vi "Positioner Control.vi"(6 "control_move_length":i64, 7 "control_positioner_reference":refnum<class "SA_CTL.lvclass">, 8 "mode":string, 9 "index":i64, 10 "control_move_direction":string, 11 "control_request":string) -> (0 "indicator_positioner_ismoving_y":bool, 1 "indicator_positioner_ismoving_x":bool, 2 "indicator_positioner_status":bool, 3 "indicator_positioner_position":cluster{"x":i64, "y":i64, "z":i64}, 4 "indicator_positioner_ismoving_z":bool, 5 "indicator_positioner_reference":refnum<class "SA_CTL.lvclass">)   [LabVIEW 2020]
uses:
  <vilib>/SmarAct/SmarActCTL/SA_CTL.lvclass
panel:
  out "error out 4":errorcluster
  out "error out 3":errorcluster
  out "error out 2":errorcluster
  out "error out":errorcluster
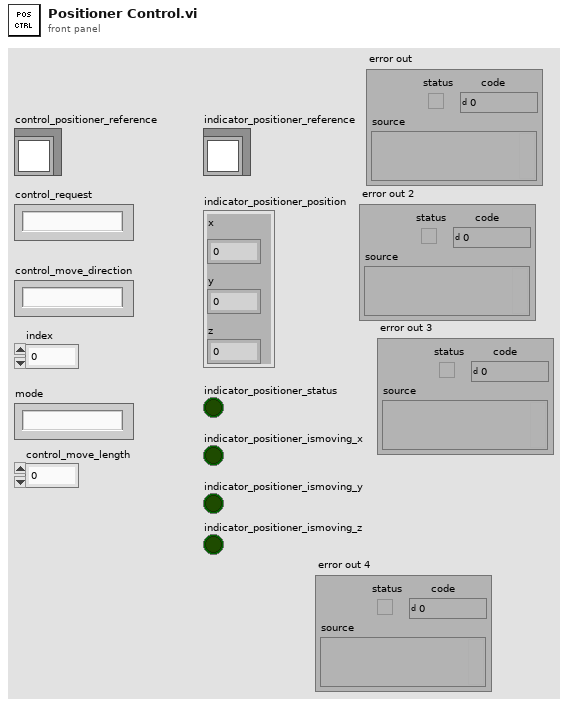
[diagram p1: front panel]
types:
  T1 = cluster{"Position":i64, "Position":i64, "Position":i64}
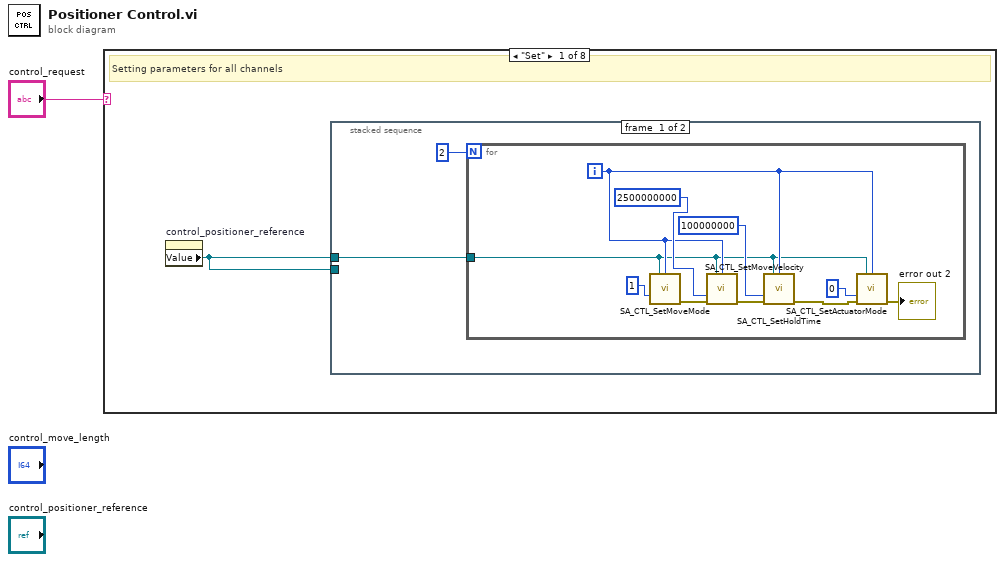
[diagram p0: block diagram]
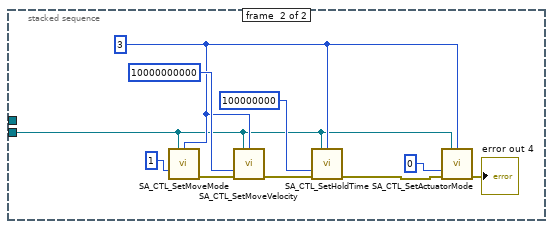
[diagram p2: hidden frame]
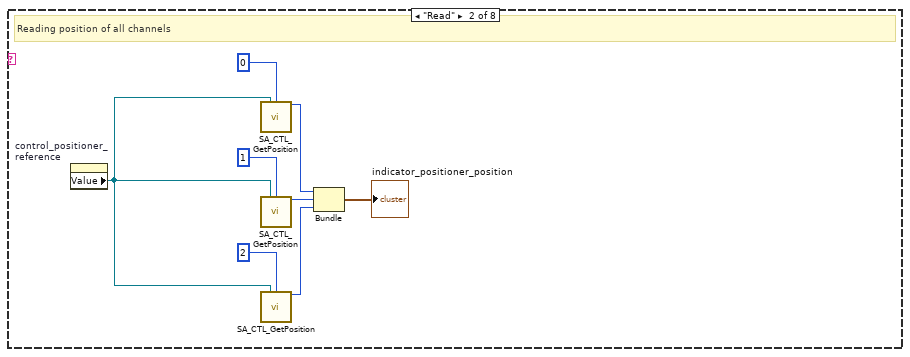
[diagram p3: hidden frame]
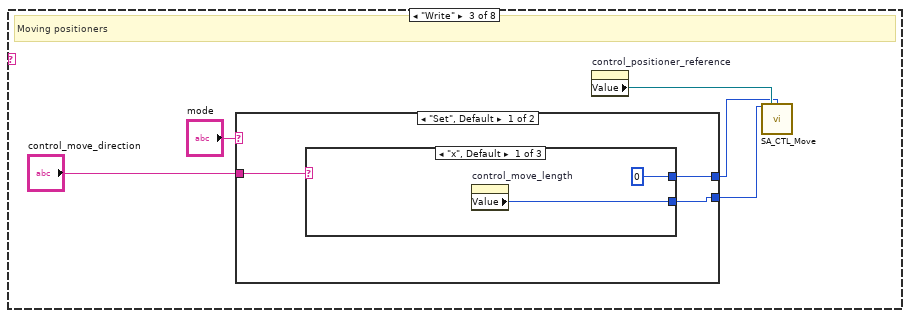
[diagram p4: hidden frame]
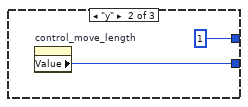
[diagram p5: hidden frame]
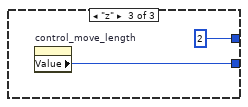
[diagram p6: hidden frame]
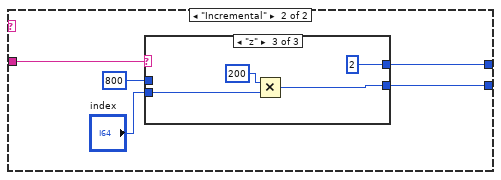
[diagram p7: hidden frame]
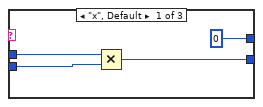
[diagram p8: hidden frame]
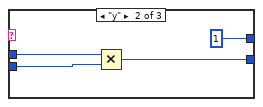
[diagram p9: hidden frame]
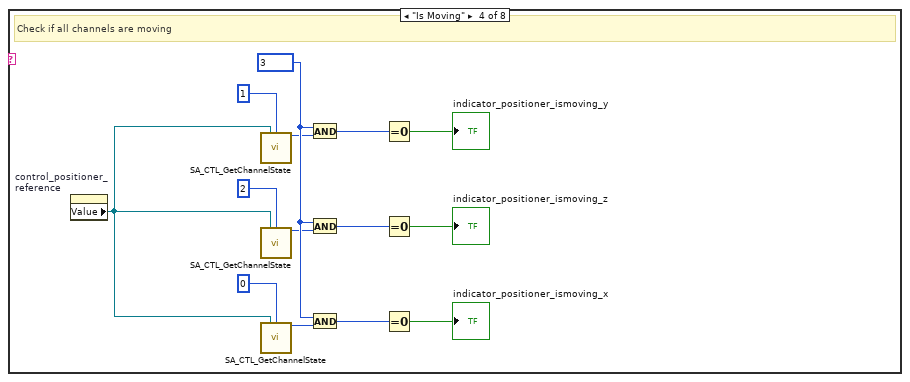
[diagram p10: hidden frame]
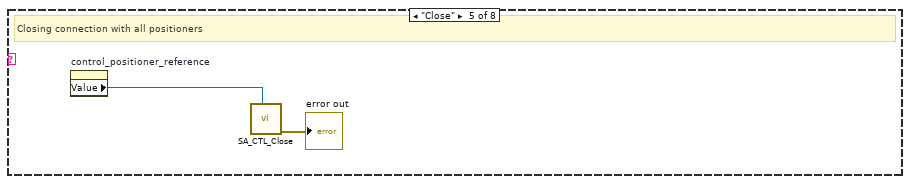
[diagram p11: hidden frame]
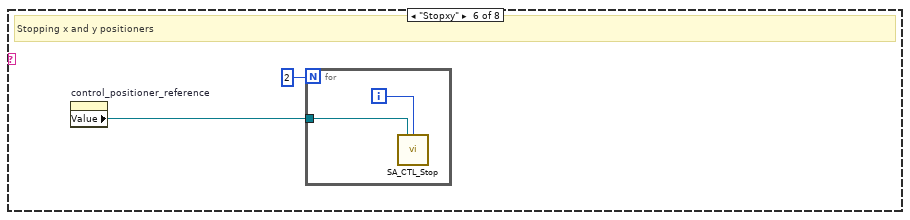
[diagram p12: hidden frame]
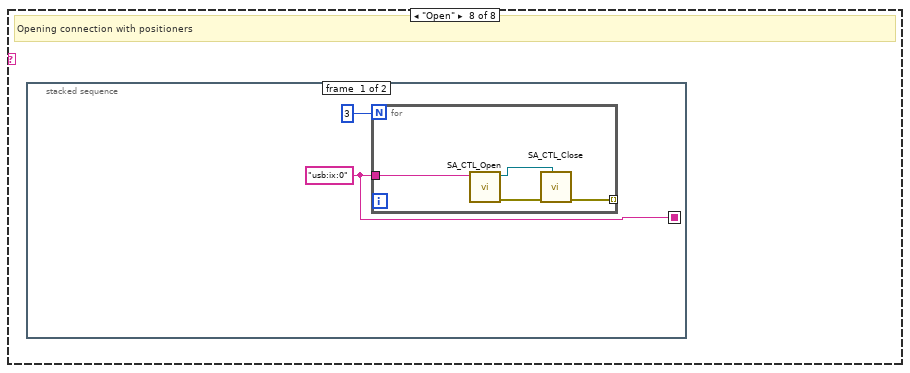
[diagram p14: hidden frame]
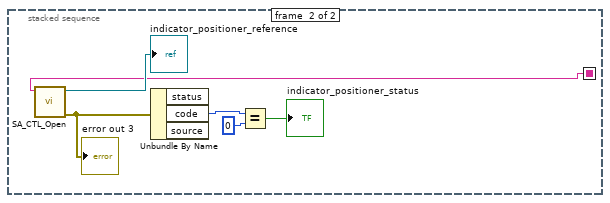
[diagram p15: hidden frame]
diagram:
  n1 = case shown="\"Set\"" "control_request" {
    frame "Set" {
      # "Setting parameters for all channels"
      n2 = property on="control_positioner_reference" class="LVClassControl (strict)"() -> ("Value"=w2:refnum<class "SA_CTL.lvclass">)  [unwired: 2 in, 2 out]
      n3 = stacked-sequence {
        tunnel: w2 -> [w3 _]
        tunnel: w2 -> [_ w16]
        frame #0 {
          n4 = for {
            N: 2 -> [_]
            tunnel: w3 -> [w5]
            i -> [w6]
            n5 = call <vilib>:"SA_CTL_SetMoveMode.vi"("SA_CTL_Handle"=w5, "channel"=w6, "MoveMode"=1) -> ("error out"=w12:errorcluster)  [unwired: 12 in]
            n6 = call <vilib>:"SA_CTL_SetMoveVelocity.vi"("SA_CTL_Handle"=w5, "channel"=w6, "MoveVelocity"=i64 2500000000 ("FindReferenceVelocity"), "error in (no error)"=w12) -> ("error out"=w11:errorcluster)  [unwired: 11 in]
            n7 = call <vilib>:"SA_CTL_SetHoldTime.vi"("SA_CTL_Handle"=w5, "channel"=w6, "HoldTime"=100000000, "error in (no error)"=w11) -> ("error out"=w9:errorcluster)  [unwired: 11 in]
            n8 = call <vilib>:"SA_CTL_SetActuatorMode.vi"("SA_CTL_Handle"=w5, "channel"=w6, "ActuatorMode"=0, "error in (no error)"=w9) -> ("error out"=→"error out 2":errorcluster)  [unwired: 11 in]
          }
        }
        frame #1 {
          w17 = 3 ("MoveMode")
          n9 = call <vilib>:"SA_CTL_SetMoveMode.vi"("SA_CTL_Handle"=w16, "channel"=w17, "MoveMode"=1) -> ("error out"=w22:errorcluster)  [unwired: 12 in]
          n10 = call <vilib>:"SA_CTL_SetMoveVelocity.vi"("SA_CTL_Handle"=w16, "channel"=w17, "MoveVelocity"=i64 10000000000 ("FindReferenceVelocity"), "error in (no error)"=w22) -> ("error out"=w21:errorcluster)  [unwired: 11 in]
          n11 = call <vilib>:"SA_CTL_SetHoldTime.vi"("SA_CTL_Handle"=w16, "channel"=w17, "HoldTime"=100000000, "error in (no error)"=w21) -> ("error out"=w19:errorcluster)  [unwired: 11 in]
          n12 = call <vilib>:"SA_CTL_SetActuatorMode.vi"("SA_CTL_Handle"=w16, "channel"=w17, "ActuatorMode"=0, "error in (no error)"=w19) -> ("error out"=→"error out 4":errorcluster)  [unwired: 11 in]
        }
      }
    }
    frame "Read" {
      # "Reading position of all channels"
      n13 = property on="control_positioner_reference" class="LVClassControl (strict)"() -> ("Value"=w32:refnum<class "SA_CTL.lvclass">)  [unwired: 2 in, 2 out]
      n14 = call <vilib>:"SA_CTL_GetPosition.vi"("SA_CTL_Handle"=w32, "channel"=i8 0) -> ("Position"=w28:i64)  [unwired: 12 in, 1 out]
      n15 = call <vilib>:"SA_CTL_GetPosition.vi"("SA_CTL_Handle"=w32, "channel"=i8 1) -> ("Position"=w27:i64)  [unwired: 12 in, 1 out]
      n16 = call <vilib>:"SA_CTL_GetPosition.vi"("SA_CTL_Handle"=w32, "channel"=i8 2) -> ("Position"=w26:i64)  [unwired: 12 in, 1 out]
      n17 = Bundle("Position"=w28, "Position"=w27, "Position"=w26) -> (→"indicator_positioner_position":T1)  [unwired: 1 in]
    }
    frame "Write" {
      # "Moving positioners"
      n18 = case shown="\"Set\", Default" "mode" {
        tunnel: "control_move_direction" -> [w40 w51]
        tunnel: [w38 w49] -> w35
        tunnel: [w39 w48] -> w34
        frame "Set", Default {
          n19 = case shown="\"x\", Default" w40 {
            tunnel: [w41 w43 w45] -> w38
            tunnel: [i8 0 ("channel") i8 1 ("channel") i8 2 ("channel")] -> w39
            frame "x", Default {
              n20 = property on="control_move_length" class="DigNum (strict)"() -> ("Value"=w41:i64)  [unwired: 2 in, 2 out]
            }
            frame "y" {
              n21 = property on="control_move_length" class="DigNum (strict)"() -> ("Value"=w43:i64)  [unwired: 2 in, 2 out]
            }
            frame "z" {
              n22 = property on="control_move_length" class="DigNum (strict)"() -> ("Value"=w45:i64)  [unwired: 2 in, 2 out]
            }
          }
        }
        frame "Incremental" {
          n23 = case shown="\"z\"" w51 {
            tunnel: "index" -> [w55 w59 w63]
            tunnel: [w54 w57 w61] -> w49
            tunnel: [i8 0 ("channel") i8 1 ("channel") i8 2 ("channel")] -> w48
            tunnel: i64 800 ("moveValue") -> [w52 w56 _]
            frame "x", Default {
              n24 = Multiply(x=w52, y=w55) -> (x*y=w54:i64)
            }
            frame "y" {
              n25 = Multiply(x=w56, y=w59) -> (x*y=w57:i64)
            }
            frame "z" {
              n26 = Multiply(x=i64 200, y=w63) -> (x*y=w61:i64)
            }
          }
        }
      }
      n27 = property on="control_positioner_reference" class="LVClassControl (strict)"() -> ("Value"=w36:refnum<class "SA_CTL.lvclass">)  [unwired: 2 in, 2 out]
      n28 = call <vilib>:"SA_CTL_Move.vi"("moveValue"=w35, "SA_CTL_Handle"=w36, "channel"=w34) -> ()  [unwired: 12 in, 1 out]
    }
    frame "Is Moving" {
      w70 = 3 ("Mask")
      # "Check if all channels are moving"
      n29 = property on="control_positioner_reference" class="LVClassControl (strict)"() -> ("Value"=w74:refnum<class "SA_CTL.lvclass">)  [unwired: 2 in, 2 out]
      n30 = call <vilib>:"SA_CTL_GetChannelState.vi"("SA_CTL_Handle"=w74, "channel"=i8 1) -> ("ChannelState"=w68:i32)  [unwired: 12 in, 1 out]
      n31 = call <vilib>:"SA_CTL_GetChannelState.vi"("SA_CTL_Handle"=w74, "channel"=i8 2) -> ("ChannelState"=w67:i32)  [unwired: 12 in, 1 out]
      n32 = call <vilib>:"SA_CTL_GetChannelState.vi"("SA_CTL_Handle"=w74, "channel"=i8 0) -> ("ChannelState"=w69:i32)  [unwired: 12 in, 1 out]
      n33 = And(x=w70, y=w68) -> (x .and. y?=w72:i32)
      n34 = And(x=w70, y=w67) -> (x .and. y?=w71:i32)
      n35 = And(x=w70, y=w69) -> (x .and. y?=w73:i32)
      n36 = Equal To 0?(x=w72) -> (x = 0?=→"indicator_positioner_ismoving_y":bool)
      n37 = Equal To 0?(x=w71) -> (x = 0?=→"indicator_positioner_ismoving_z":bool)
      n38 = Equal To 0?(x=w73) -> (x = 0?=→"indicator_positioner_ismoving_x":bool)
    }
    frame "Close" {
      # "Closing connection with all positioners"
      n39 = property on="control_positioner_reference" class="LVClassControl (strict)"() -> ("Value"=w79:refnum<class "SA_CTL.lvclass">)  [unwired: 2 in, 2 out]
      n40 = call <vilib>:"SA_CTL_Close.vi"("SA_CTL_Handle"=w79) -> ("error out"=→"error out":errorcluster)  [unwired: 10 in]
    }
    frame "Stopxy" {
      # "Stopping x and y positioners"
      n41 = property on="control_positioner_reference" class="LVClassControl (strict)"() -> ("Value"=w81:refnum<class "SA_CTL.lvclass">)  [unwired: 2 in, 2 out]
      n42 = for {
        N: 2 -> [_]
        tunnel: w81 -> [w83]
        i -> [w82]
        n43 = call <vilib>:"SA_CTL_Stop.vi"("SA_CTL_Handle"=w83, "channel"=w82) -> ()  [unwired: 13 in, 1 out]
      }
    }
    frame "Default", Default {
    }
    frame "Open" {
      # "Opening connection with positioners"
      n44 = stacked-sequence {
        seq-local: [w84 _] -> [_ w90]
        frame #0 {
          w84 = "usb:ix:0" ("locator")
          n45 = for {
            N: 3 -> [_]
            tunnel: w84 -> [w87]
            tunnel: [w86] -> _ mode=indexing
            n46 = call <vilib>:"SA_CTL_Open.vi"("locator"=w87) -> ("error out"=w88:errorcluster, "SA_CTL_Handle"=w89:refnum<class "SA_CTL.lvclass">)  [unwired: 9 in]
            n47 = call <vilib>:"SA_CTL_Close.vi"("SA_CTL_Handle"=w89, "error in (no error)"=w88) -> ("error out"=w86:errorcluster)  [unwired: 9 in]
          }
        }
        frame #1 {
          n48 = call <vilib>:"SA_CTL_Open.vi"("locator"=w90) -> ("error out"=w93:errorcluster, "SA_CTL_Handle"=→"indicator_positioner_reference":refnum<class "SA_CTL.lvclass">)  [unwired: 9 in]
          "error out 3" <- w93
          n49 = Unbundle By Name(w93) -> ("code"=w94:i32)  [unwired: 2 out]
          n50 = Equal?(x=w94, y=0) -> (x = y?=→"indicator_positioner_status":bool)
        }
      }
    }
  }
